vi "CreateOctaFile.vi"(3 "error in":errorcluster, 4 "Memory (GB)":dbl format="%#_3g", 5 "File control":T1={"Subject ID"="", "Eye"=FALSE, "Output Path"=path "E:/test", "String"="", "String 2"=""}) -> (0 "error out":errorcluster, 1 "OCT filename out":string, 2 "OCTA refnum out":refnum<file>)   [LabVIEW 2017]
panel:
  out "Eye indicator":string
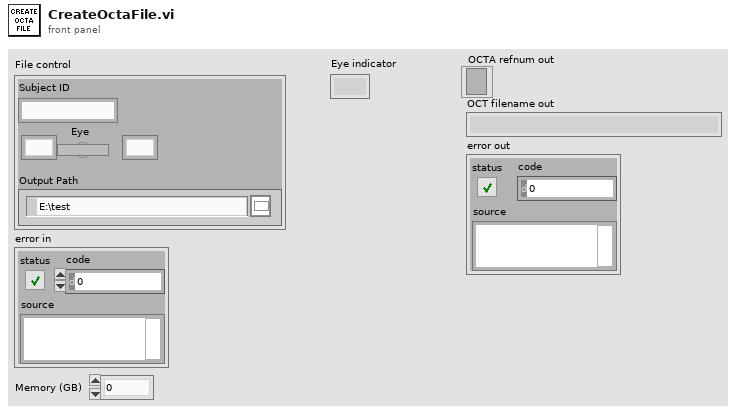
[diagram p1: front panel]
types:
  T1 = cluster{"Subject ID":string, "Eye":bool, "Output Path":path, "String":string, "String 2":string}
  T2 = enum16{"open", "replace", "create", "open or create", "replace or create", "replace or create with confirmation"}
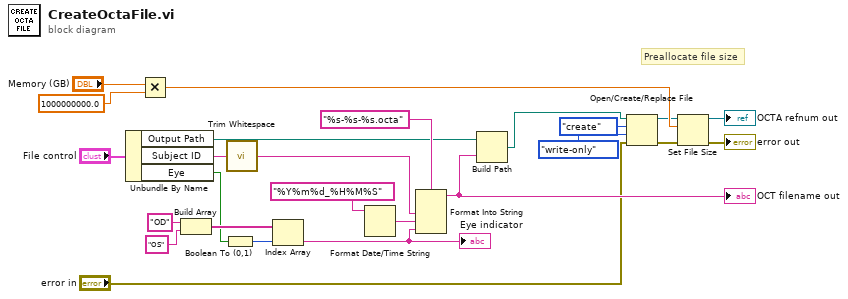
[diagram p0: block diagram]
diagram:
  # "Preallocate file size"
  n1 = Unbundle By Name("File control") -> ("Output Path"=w19:path, "Subject ID"=w15:string, "Eye"=w13:bool)
  n2 = Multiply(x="Memory (GB)", y=1000000000.0) -> (x*y=w5:dbl)
  n3 = Build Array("OD", "OS") -> (w25:string[])
  n4 = Boolean To (0,1)(Boolean=w13) -> (0, 1=w10:i16)
  n5 = call <vilib>:"Trim Whitespace.vi"("string"=w15) -> ("trimmed string"=w14:string)  [unwired: 1 in]
  n6 = Index Array(array=w25, index=w10) -> (element=w9:string)
  "Eye indicator" <- w9
  n7 = Format Date/Time String(time format string (%c)="%Y%m%d_%H%M%S") -> (date/time string=w23:string)  [unwired: 2 in]
  n8 = Format Into String(format string="%s-%s-%s.octa", w14, w23, w9) -> (resulting string=w20:string)  [unwired: 2 in, 1 out]
  "OCT filename out" <- w20
  n9 = Build Path(base path=w19, name or relative path=w20) -> (appended path=w16:path)
  n10 = Open/Create/Replace File(file path (use dialog)=w16, error in="error in", operation (0:open)=T2."create", access (0:read/write)=enum16{"read/write", "read-only", "write-only"}."write-only") -> (refnum out=w4:refnum<file>, error out=w3:errorcluster)  [unwired: 2 in, 1 out]
  n11 = Set File Size(4:w3, 6:w5, 7:w4) -> (0:→"error out":errorcluster, 3:→"OCTA refnum out":refnum<file>)
